vi "transferData2UnitFormat.vi"(4 "displayRef":T1, 5 "Data":T3[](array[typedef])) -> (2 "display":dbl[][](array[numeric]))   [LabVIEW 2010]
uses:
  types/OutputDataFormat.ctl
  types/VarableID.ctl
panel:
  out "output array 2":dbl[](array[numeric])
  out "display 2":T2
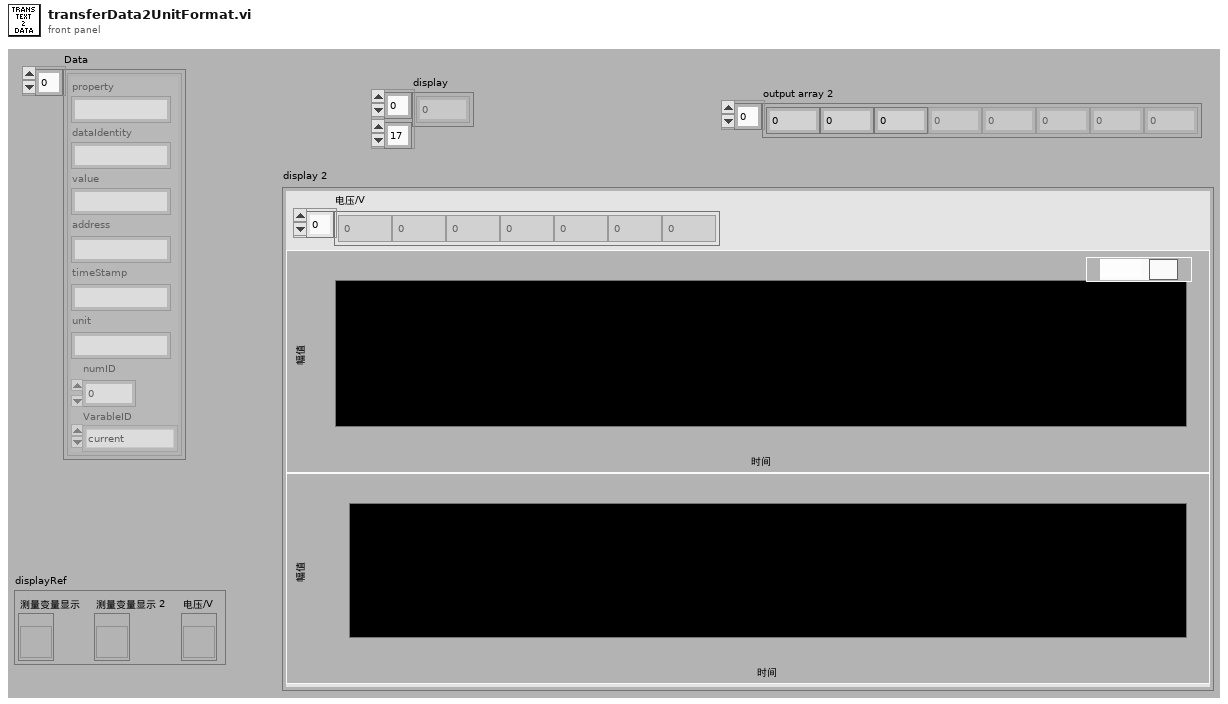
[diagram p1: front panel]
types:
  T1 = cluster{"测量变量显示":refnum<vi>, "测量变量显示 2":refnum<vi>, "电压/V":refnum<vi>}
  T2 = cluster{"测量变量显示":dbl[][], "测量变量显示 2":dbl[][], "电压/V":dbl[]}
  T3 = typedef "OutputDataFormat.ctl" = cluster{"property":string, "dataIdentity":string, "value":string, "address":string, "timeStamp":string, "unit":string, "numID":i32, "VarableID":T4}
  T4 = typedef "VarableID.ctl" = enum16{"current", "power", "PF", "voltage"}
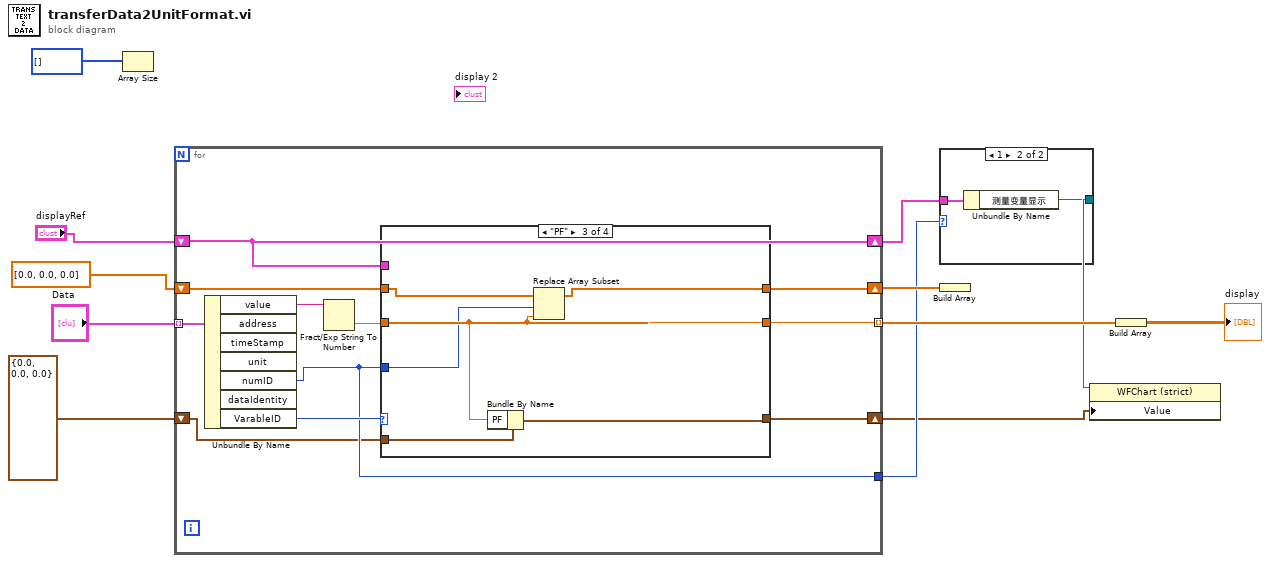
[diagram p0: block diagram]
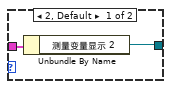
[diagram p2: hidden frame]
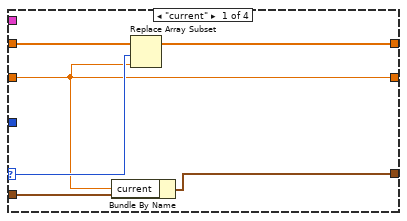
[diagram p3: hidden frame]
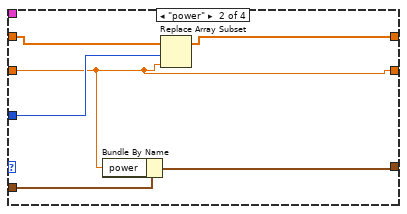
[diagram p4: hidden frame]
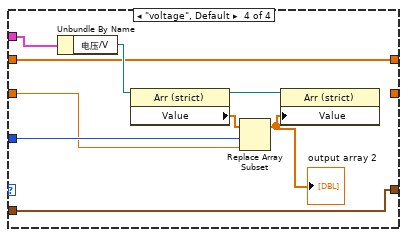
[diagram p5: hidden frame]
diagram:
  n1 = Array Size(array=i32[] []) -> ()  [unwired: 1 out]
  n2 = for {
    tunnel: "Data" -> [w23] mode=indexing
    tunnel: [w19] -> w11 mode=indexing
    shift-right: [w17] -> w8
    shift-left: dbl[] [0.0, 0.0, 0.0] -> [w18]
    tunnel: [w16] -> w6
    shift-right: [w14] -> w5
    shift-left: cluster{"current":dbl, "power":dbl, "PF":dbl} {"current"=0.0, "power"=0.0, "PF"=0.0} -> [w15]
    shift-right: [w13] -> w3
    shift-left: "displayRef" -> [w13]
    n3 = Unbundle By Name(w23) -> ("value"=w22:string, "numID"=w16:i32, "VarableID"=w21:T4)  [unwired: 4 out]
    n4 = Fract/Exp String To Number(string=w22) -> (number=w20:dbl)  [unwired: 3 in, 1 out]
    n5 = case shown="\"PF\"" w21 {
      selector: w21 -> [w28 _ _ _]
      tunnel: w16 -> [_ w33 w36 w46]
      tunnel: w13 -> [_ _ _ w45]
      tunnel: w20 -> [w25 w30 w37 w44]
      tunnel: [w25 w30 w37 _] -> w19
      tunnel: w18 -> [w29 w32 w41 w43]
      tunnel: [w27 w31 w40 w43] -> w17
      tunnel: w15 -> [w26 w35 w38 w42]
      tunnel: [w24 w34 w39 w42] -> w14
      frame "current" {
        n6 = Bundle By Name(cluster=w26, "current"=w25) -> (w24:cluster{"current":dbl, "power":dbl, "PF":dbl})
        n7 = Replace Array Subset(array=w29, new element=w25, index=w28) -> (w27:dbl[])
      }
      frame "power" {
        n8 = Bundle By Name(cluster=w35, "power"=w30) -> (w34:cluster{"current":dbl, "power":dbl, "PF":dbl})
        n9 = Replace Array Subset(array=w32, new element=w30, index=w33) -> (w31:dbl[])
      }
      frame "PF" {
        n10 = Bundle By Name(cluster=w38, "PF"=w37) -> (w39:cluster{"current":dbl, "power":dbl, "PF":dbl})
        n11 = Replace Array Subset(array=w41, new element=w37, index=w36) -> (w40:dbl[])
      }
      frame "voltage", Default {
        n12 = Unbundle By Name(w45) -> ("电压/V"=w50:refnum<vi>)
        n13 = property class="Arr (strict)"(reference=w50) -> (reference out=w47:refnum<vi>, "Value"=w48:dbl[])  [unwired: 1 in, 1 out]
        n14 = Replace Array Subset(array=w48, new element=w44, index=w46) -> (w49:dbl[])
        "output array 2" <- w49
        n15 = property class="Arr (strict)"(reference=w47, "Value"=w49) -> ()  [unwired: 1 in, 2 out]
      }
    }
  }
  n16 = case shown="1" w6 {
    tunnel: w3 -> [w52 w54]
    tunnel: [w51 w53] -> w7
    frame 2, Default {
      n17 = Unbundle By Name(w52) -> ("测量变量显示 2"=w51:refnum<vi>)
    }
    frame 1 {
      n18 = Unbundle By Name(w54) -> ("测量变量显示"=w53:refnum<vi>)
    }
  }
  n19 = Build Array(w8) -> ()  [unwired: 1 out]
  n20 = property class="WFChart (strict)"(reference=w7, "Value"=w5) -> ()  [unwired: 1 in, 2 out]
  n21 = Build Array(w11) -> (→"display":dbl[][])
